vi "subGetDiComponentsRootRef.vi"(8 "error in (no error)":errorcluster, 11 "Refnum in":refnum<k20>) -> (0 "error out":errorcluster, 1 "DIComponents ref":refnum<k20>, 3 "Refnum out":refnum<k20>)   [LabVIEW 2020, in "DefaultExtensions.lvlib" / "CDefaultRuleFileParser.lvclass"]
uses:
  CDefaultRuleFileParser.lvclass
  <resource>/objmgr/DOMUserDefRef.rc
  <vilib>/xml/NI_XML.lvlib
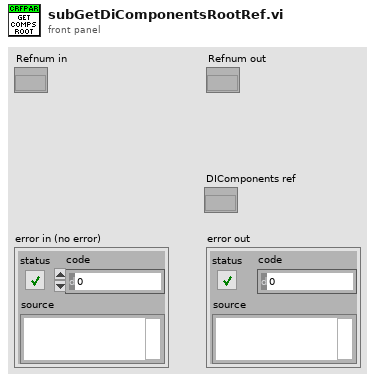
[diagram p1: front panel]
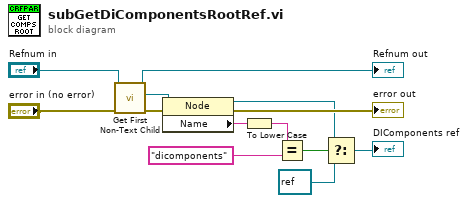
[diagram p0: block diagram]
diagram:
  n1 = call <vilib>:"Get First Non-Text Child.vi"("error in (no error)"="error in (no error)", "node in"="Refnum in") -> ("error out"=w8:errorcluster, "child node"=w11:refnum<k20>, "node out"=→"Refnum out":refnum<k20>)  [unwired: 6 in, 1 out]
  n2 = property class="Node"(reference=w11, error in=w8) -> (reference out=w3:refnum<k20>, error out=→"error out":errorcluster, "Name"=w10:string)
  n3 = To Lower Case(string=w10) -> (all lower case string=w6:string)
  n4 = Equal?(x=w6, y="dicomponents" ("XPath expression")) -> (x = y?=w4:bool)
  n5 = Select(t=w3, s=w4, f=refnum<k20> refnum) -> (s? t:f=→"DIComponents ref":refnum<k20>)
